vi "ID to Item.vi"(10 "ID":string) -> (2 "Item":T1)   [LabVIEW 2015, in "Read-Write-Signals.xnode"]
uses:
  Read-Write-Signals.xnode
  Read-Write-Signals Item.ctl
  Read-Write-Signals Sub Item.ctl
  Read-Write-Signals Sub Item Type.ctl
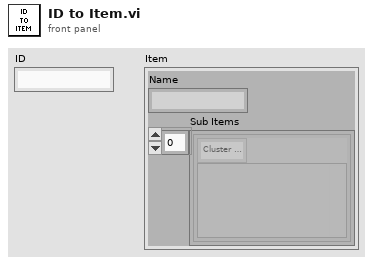
[diagram p1: front panel]
types:
  T1 = typedef "Read-Write-Signals Item.ctl" = cluster{"Name":string, "Sub Items":T2[]}
  T2 = typedef "Read-Write-Signals Sub Item.ctl" = cluster{"Type":T3, "Value":variant}
  T3 = typedef "Read-Write-Signals Sub Item Type.ctl" = enum8{"Cluster Element", "Array Element", "Subarray"}
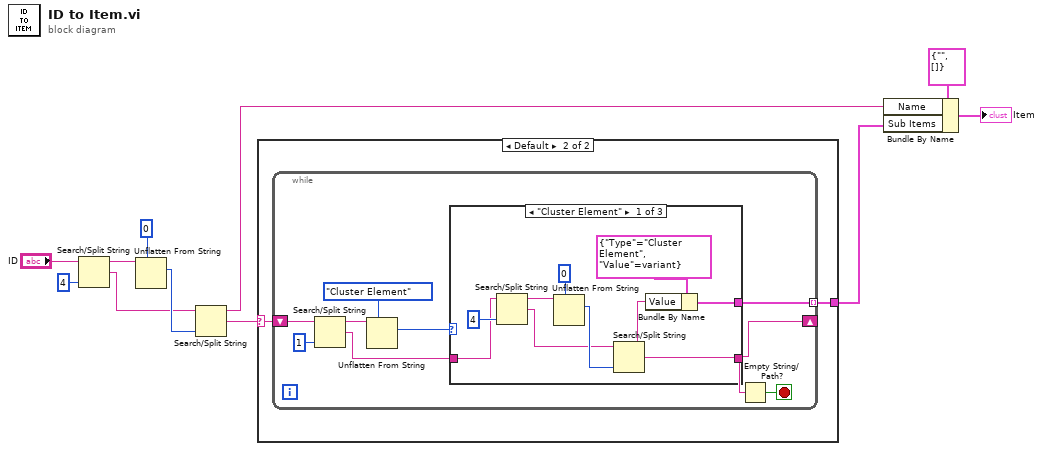
[diagram p0: block diagram]
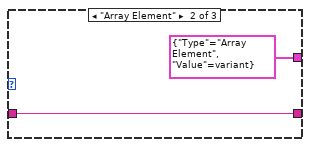
[diagram p3: hidden frame]
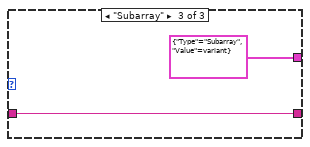
[diagram p4: hidden frame]
diagram:
  n1 = Search/Split String(string="ID", offset (0)=4) -> (substring before match=w4:string, match + rest of string=w6:string)  [unwired: 1 in, 1 out]
  n2 = Unflatten From String(type=0, binary string=w4) -> (value=w7:i32)  [unwired: 3 in, 2 out]
  n3 = Search/Split String(string=w6, offset (0)=w7) -> (substring before match=w1:string, match + rest of string=w8:string)  [unwired: 1 in, 1 out]
  n4 = case shown="Default" w8 {
    selector: w8 -> [_ w13]
    tunnel: [_ w12] -> w10
    frame "" {
    }
    frame Default {
      n5 = while {
        shift-right: [w15] -> _
        shift-left: w13 -> [w21]
        tunnel: [w14] -> w12 mode=indexing
        stop <- w22 stop-if-true
        n6 = Search/Split String(string=w21, offset (0)=1) -> (substring before match=w19:string, match + rest of string=w17:string)  [unwired: 1 in, 1 out]
        n7 = Unflatten From String(type=Read-Write-Signals_Sub_Item_Type."Cluster Element" ("Type"), binary string=w19) -> (value=w16:T3)  [unwired: 3 in, 2 out]
        n8 = case shown="\"Cluster Element\"" w16 {
          tunnel: w17 -> [w27 w34 w36]
          tunnel: [w25 w34 w36] -> w15
          tunnel: [w24 T2 {"Type"=enum."Array Element", "Value"=variant} ("Sub Items") T2 {"Type"=enum."Subarray", "Value"=variant} ("Sub Items")] -> w14
          frame "Cluster Element" {
            n9 = Search/Split String(string=w27, offset (0)=4) -> (substring before match=w29:string, match + rest of string=w31:string)  [unwired: 1 in, 1 out]
            n10 = Unflatten From String(type=0, binary string=w29) -> (value=w32:i32)  [unwired: 3 in, 2 out]
            n11 = Search/Split String(string=w31, offset (0)=w32) -> (substring before match=w23:string, match + rest of string=w25:string)  [unwired: 1 in, 1 out]
            n12 = Bundle By Name(cluster=T2 {"Type"=enum."Cluster Element", "Value"=variant} ("Sub Items"), "Value"=w23) -> (w24:T2)
          }
          frame "Array Element" {
          }
          frame "Subarray" {
          }
        }
        n13 = Empty String/Path?(string/path=w15) -> (empty?=w22:bool)
      }
    }
  }
  n14 = Bundle By Name(cluster=T1 {"Name"="", "Sub Items"=[]} ("Item"), "Name"=w1, "Sub Items"=w10) -> (→"Item":T1)
